vi "Actor Core.vi"(8 "error in":errorcluster, 11 "My Application":refnum<class "State Pattern UI.lvclass">) -> (0 "error out":errorcluster, 3 "Actor out":refnum<class "Actor.lvclass">)   [LabVIEW 2020, in "State Pattern UI.lvlib" / "State Pattern UI.lvclass"]
doc: "This is Actor Core.vi, the main message handling loop for Actors. An actor usually just sits in this loop and processes messages as they arrive. Any error returned by the message Do.vi call will stop the loop, with error code 43 as the canonical signal to stop with no error sent to caller. Descendants may override that in Handle Error.vi."
uses:
  State Pattern UI.lvclass
  C:/Program Files (x86)/National Instruments/LabVIEW 2020/vi.lib/ActorFramework/Actor/Actor.lvclass
  <vilib>/ActorFramework/Actor/Actor.lvclass
  Process States/Idle/Idle.lvclass
  <vilib>/ActorFramework/Actor/Actor.lvclass/Actor.ctl
  <vilib>/ActorFramework/Message Enqueuer/Message Enqueuer.lvclass/Message Enqueuer.ctl
  State Pattern UI.lvclass/State Pattern UI.ctl
  <vilib>/ActorFramework/Message Enqueuer/Init from Existing Queue.vi
  <vilib>/ActorFramework/Message Enqueuer/Enqueue.vi
  <vilib>/ActorFramework/Stop Msg/Stop Msg.lvclass
  C:/Program Files (x86)/National Instruments/LabVIEW 2020/vi.lib/ActorFramework/Message/Message.lvclass
  Process States/Process State Messages/Go to Running Msg/Go to Running Msg.lvclass
  Process States/Process State Messages/Go to Idle Msg/Go to Idle Msg.lvclass
  Process States/Process State Messages/Request Update from Process Msg/Request Update from Process Msg.lvclass
  <vilib>/ActorFramework/Message Priority Queue/Priority Enqueue.vi
  <vilib>/ActorFramework/Message Enqueuer/Message Enqueuer.lvclass
panel:
  in  "Message to State 3":bool
  in  "Message to State 2":bool
  in  "stop signal":bool
  out "Event Log":string
  in  "DNL_Stop":bool
  in  "Message to State":bool
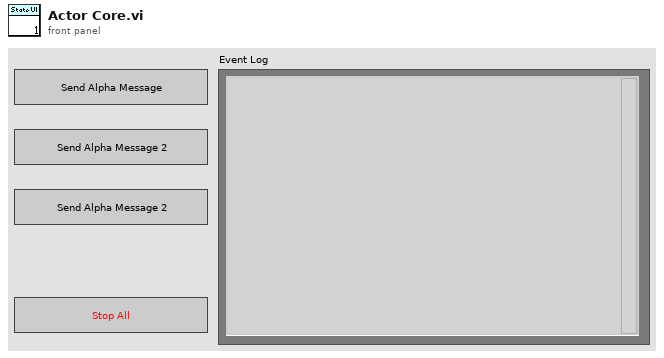
[diagram p1: front panel]
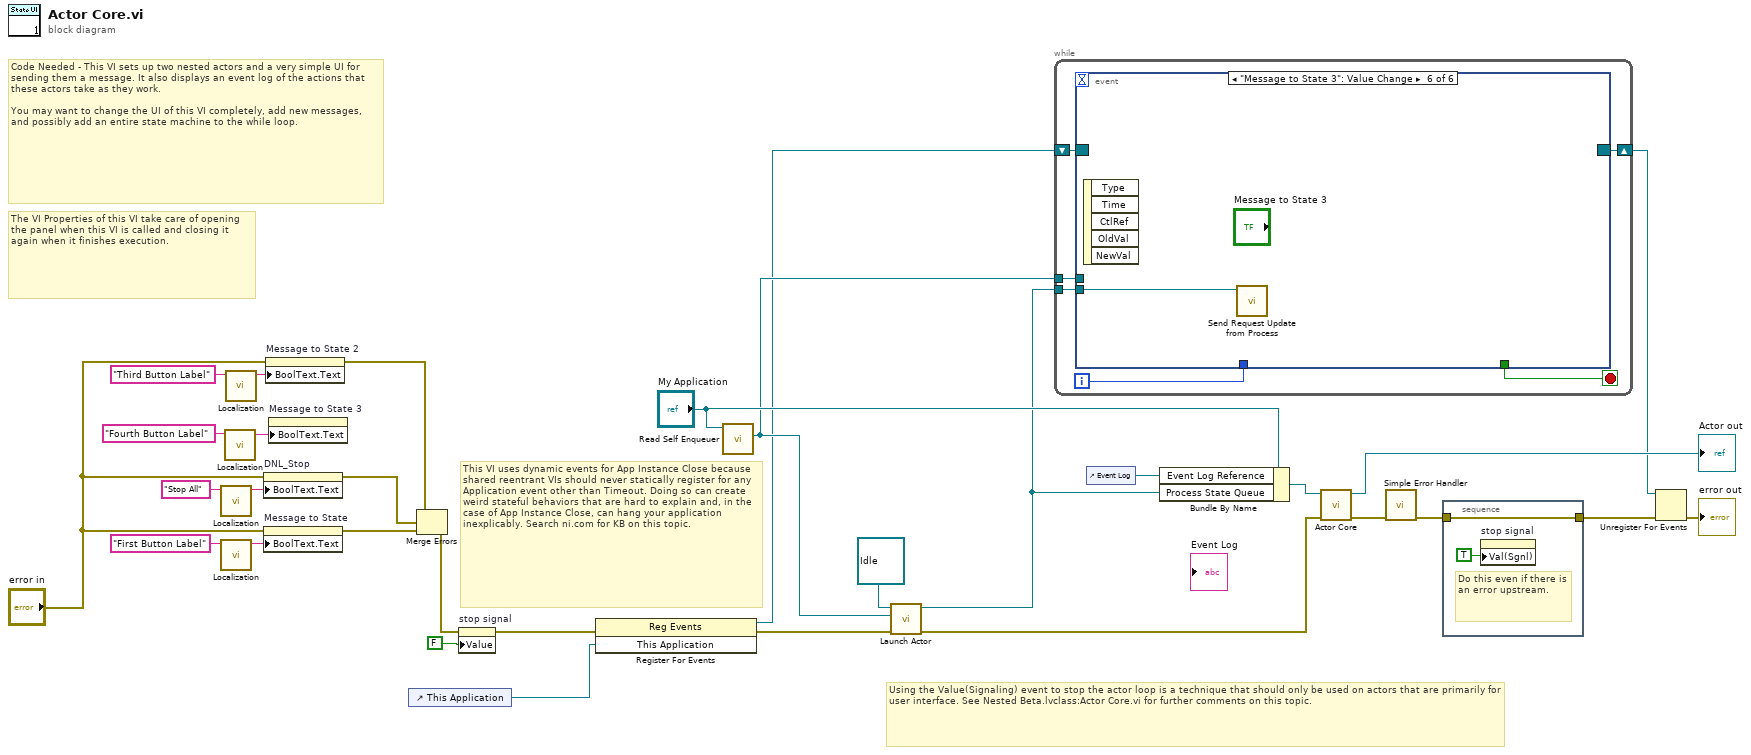
[diagram p0: block diagram]
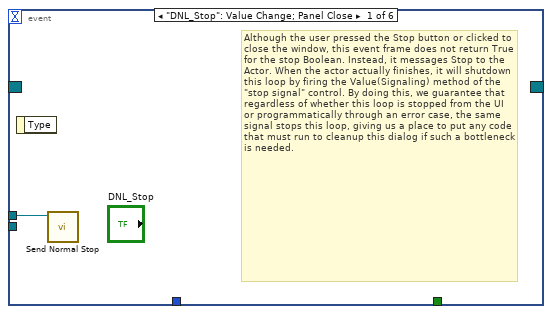
[diagram p2: hidden frame]
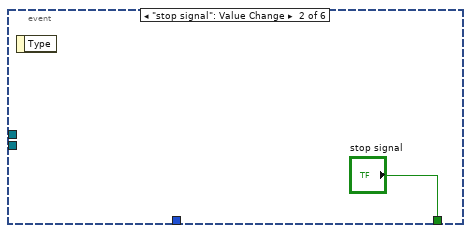
[diagram p3: hidden frame]
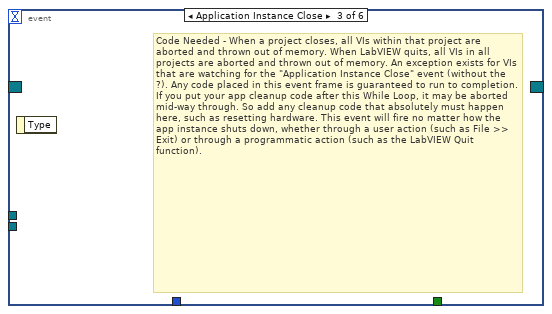
[diagram p4: hidden frame]
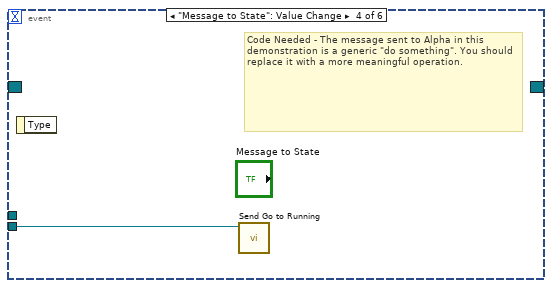
[diagram p5: hidden frame]
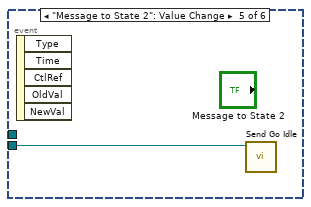
[diagram p6: hidden frame]
diagram:
  # "This VI uses dynamic events for App Instance Close because shared reentrant VIs should never statically register for any Application event other than Timeout. Doing so can create weird stateful behaviors that are hard to explain and, in the case of App Instance Close, can hang your application inexplicably. Search ni.com for KB on this topic."
  # "The VI Properties of this VI take care of opening the panel when this VI is called and closing it again when it finishes execution."
  # "Using the Value(Signaling) event to stop the actor loop is a technique that should only be used on actors that are primarily for user interface. See Nested Beta.lvclass:Actor Core.vi for further comments on this topic."
  # "Code Needed - This VI sets up two nested actors and a very simple UI for sending them a message. It also displays an event log of the actions that these actors take as they work. \n\nYou may want to change the UI of this VI completely, add new messages, and possibly add an entire state machine to the while loop."
  n1 = call "Localization.vi"("Unlocalized"="Stop All") -> ("Localized"=w21:string)  [unwired: 10 in]
  n2 = call "Localization.vi"("Unlocalized"="First Button Label") -> ("Localized"=w23:string)  [unwired: 10 in]
  n3 = call "Localization.vi"("Unlocalized"="Fourth Button Label") -> ("Localized"=w1:string)  [unwired: 10 in]
  n4 = call "Localization.vi"("Unlocalized"="Third Button Label") -> ("Localized"=w4:string)  [unwired: 10 in]
  n5 = property on="DNL_Stop" class="Bool"(error in="error in", "BoolText.Text"=w21) -> (error out=w20:errorcluster)  [unwired: 1 in, 1 out]
  n6 = property on="Message to State" class="Bool"(error in="error in", "BoolText.Text"=w23) -> (error out=w19:errorcluster)  [unwired: 1 in, 1 out]
  n7 = property on="Message to State 2" class="Bool"(error in="error in", "BoolText.Text"=w4) -> (error out=w6:errorcluster)  [unwired: 1 in, 1 out]
  n8 = property on="Message to State 3" class="Bool"("BoolText.Text"=w1) -> ()  [unwired: 2 in, 2 out]
  n9 = control-ref of="This Application"() -> (w9:refnum<vi>)
  n10 = Merge Errors(w6, w20, w19) -> (w18:errorcluster)
  n11 = property on="stop signal" class="Bool (strict)"(error in=w18, "Value"=FALSE ("stop")) -> (error out=w11:errorcluster)  [unwired: 1 in, 1 out]
  n12 = register-events(error in=w11, w9) -> (reference out=w15:refnum<event-registration>, error out=w10:errorcluster)  [unwired: 1 in]
  n13 = call <vilib>:"Read Self Enqueuer.vi"("Actor"="My Application") -> ("Self Enqueuer"=w26:refnum<class "Message Enqueuer.lvclass">)  [unwired: 10 in]
  n14 = call <vilib>:"Launch Actor.vi"("error in (no error)"=w10, "Actor-to-Caller Enqueuer"=w26, "Actor"=refnum<class "Idle.lvclass"> refnum ("Process States.lvlib:Ilde.lvclass")) -> ("error out"=w30:errorcluster, "Caller-To-Actor Enqueuer"=w8:refnum<class "Message Enqueuer.lvclass">)  [unwired: 7 in]
  n15 = while {
    tunnel: w26 -> [w37]
    tunnel: w8 -> [w36]
    shift-right: [w32] -> w14
    shift-left: w15 -> [w33]
    i -> [w34]
    stop <- w35 stop-if-true
    n16 = event shown="[5] \"Message to State 3\": Value Change" {
      selector: w33 -> [_ _ _ _ _ _]
      dyn-events: [_ _ _ _ _ _] -> w32
      timeout: _ -> [_ _ _ _ _ _]
      tunnel: w37 -> [w38 _ _ _ _ _]
      tunnel: w36 -> [_ _ _ w40 w41 w42]
      tunnel: [_ "stop signal" _ _ _ _] -> w35
      tunnel: w34 -> [_ _ _ _ _ _]
      event "DNL_Stop": Value Change; Panel Close {
        # "Although the user pressed the Stop button or clicked to close the window, this event frame does not return True for the stop Boolean. Instead, it messages Stop to the Actor. When the actor actually finishes, it will shutdown this loop by firing the Value(Signaling) method of the \"stop signal\" control. By doing this, we guarantee that regardless of whether this loop is stopped from the UI or programmatically through an error case, the same signal stops this loop, giving us a place to put any code that must run to cleanup this dialog if such a bottleneck is needed."
        n17 = event-data() -> ()  [unwired: 1 in, 1 out]
        n18 = call <vilib>:"Send Normal Stop.vi"("Message Enqueuer"=w38) -> ()  [unwired: 10 in, 1 out]
      }
      event "stop signal": Value Change {
        n19 = event-data() -> ()  [unwired: 1 in, 1 out]
      }
      event Application Instance Close {
        # "Code Needed - When a project closes, all VIs within that project are aborted and thrown out of memory. When LabVIEW quits, all VIs in all projects are aborted and thrown out of memory. An exception exists for VIs that are watching for the \"Application Instance Close\" event (without the ?). Any code placed in this event frame is guaranteed to run to completion. If you put your app cleanup code after this While Loop, it may be aborted mid-way through. So add any cleanup code that absolutely must happen here, such as resetting hardware. This event will fire no matter how the app instance shuts down, whether through a user action (such as File >> Exit) or through a programmatic action (such as the LabVIEW Quit function)."
        n20 = event-data() -> ()  [unwired: 1 in, 1 out]
      }
      event "Message to State": Value Change {
        # "Code Needed - The message sent to Alpha in this demonstration is a generic \"do something\". You should replace it with a more meaningful operation."
        n21 = event-data() -> ()  [unwired: 1 in, 1 out]
        n22 = call "Send Go to Running.vi"("Message Enqueuer"=w40) -> ()  [unwired: 9 in, 2 out]
      }
      event "Message to State 2": Value Change {
        n23 = event-data() -> ()  [unwired: 1 in, 5 out]
        n24 = call "Send Go Idle.vi"("Message Enqueuer"=w41) -> ()  [unwired: 9 in, 2 out]
      }
      event "Message to State 3": Value Change {
        n25 = event-data() -> ()  [unwired: 1 in, 5 out]
        n26 = call "Send Request Update from Process.vi"("Message Enqueuer"=w42) -> ()  [unwired: 9 in, 2 out]
      }
    }
  }
  n27 = control-ref of="Event Log"() -> (w27:refnum<vi>)
  n28 = Bundle By Name(cluster="My Application", "Event Log Reference"=w27, "Process State Queue"=w8) -> (w28:refnum<class "State Pattern UI.lvclass">)
  n29 = call-parent "Actor Core.vi"("error in"=w30, "Actor in"=w28) -> ("error out"=w17:errorcluster, "Actor out"=→"Actor out":refnum<class "Actor.lvclass">)  [unwired: 8 in]
  n30 = call <vilib>:"Simple Error Handler.vi"("error in (no error)"=w17) -> ("error out"=w16:errorcluster)  [unwired: 4 in, 4 out]
  n31 = stacked-sequence {
    tunnel: [w43] -> w13
    tunnel: w16 -> [w43]
    frame #0 {
      # "Do this even if there is an error upstream."
      n32 = property on="stop signal" class="Bool (strict)"("Val(Sgnl)"=TRUE ("stop")) -> ()  [unwired: 2 in, 2 out]
    }
  }
  n33 = Unregister For Events(event registration refnum=w14, error in=w13) -> (error out=→"error out":errorcluster)
